vi "Ramp Trans Down.vi"(9 "Time (ms)":u32=500, 10 "Transparency":u32, 11 "VI Ref In":refnum<vi>) -> (3 "VI Ref Out":refnum<vi>)   [LabVIEW 2016, in "Rectangle Mask.lvclass"]
uses:
  Classes/Rectangle Mask/Rectangle Mask.lvclass
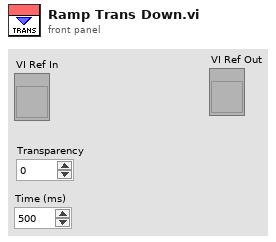
[diagram p1: front panel]
types:
  T1 = enum32{"Invalid", "Standard", "Closed", "Hidden", "Minimized", "Maximized"}
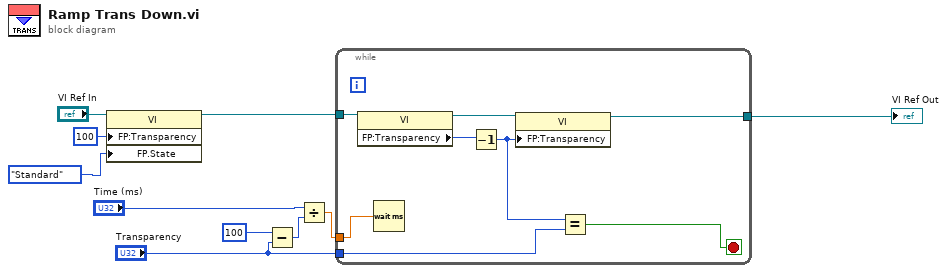
[diagram p0: block diagram]
diagram:
  n1 = property class="VI"(reference="VI Ref In", "FP:Transparency"=u8 100 ("Front Panel Window:Transparency"), "FP.State"=T1."Standard" ("Front Panel Window:State")) -> (reference out=w4:refnum<vi>)  [unwired: 1 in, 1 out]
  n2 = Subtract(x=u32 100, y="Transparency") -> (x-y=w8:u32)
  n3 = Divide(x="Time (ms)", y=w8) -> (x/y=w10:dbl)
  n4 = while {
    tunnel: w10 -> [w18]
    tunnel: w4 -> [w17]
    tunnel: [w12] -> w6
    tunnel: "Transparency" -> [w11]
    stop <- w13 stop-if-true
    n5 = property class="VI"(reference=w17) -> (reference out=w15:refnum<vi>, "FP:Transparency"=w16:u8)  [unwired: 1 in, 1 out]
    n6 = Wait (ms)(milliseconds to wait=w18) -> ()  [unwired: 1 out]
    n7 = Decrement(x=w16) -> (x-1=w14:u8)
    n8 = property class="VI"(reference=w15, "FP:Transparency"=w14) -> (reference out=w12:refnum<vi>)  [unwired: 1 in, 1 out]
    n9 = Equal?(x=w14, y=w11) -> (x = y?=w13:bool)
  }
  "VI Ref Out" <- w6
